vi "TagMetadataToImage.vi"(8 "error in (no error)":errorcluster, 10 "Image In":T1, 11 "LaserController in":refnum<class "LaserController.lvclass">) -> (0 "error out":errorcluster, 2 "Image Out":T1, 3 "LaserController out":refnum<class "LaserController.lvclass">)   [LabVIEW 2020, in "LaserController.lvlib" / "LaserController.lvclass"]
uses:
  LaserController.lvclass
  <vilib>/vision/Image Controls.llb/IMAQ Image.ctl
  LaserController.lvclass/LaserController.ctl
  Model/Hardware Abstraction Layer/Component/GenericActor/GenericActor/GenericController.lvclass
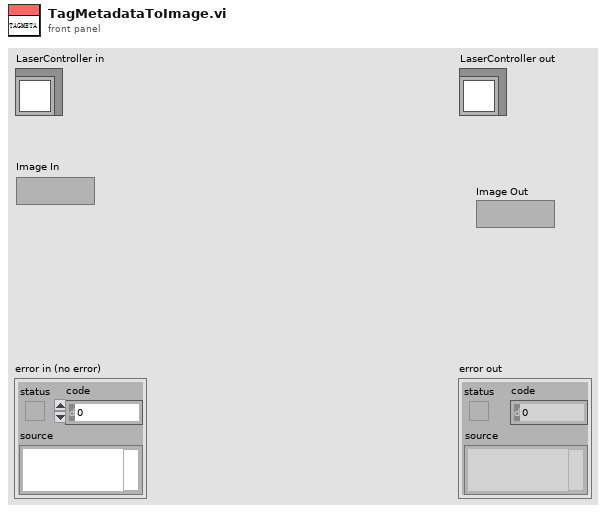
[diagram p1: front panel]
types:
  T1 = typedef "IMAQ Image.ctl" = refnum<image>
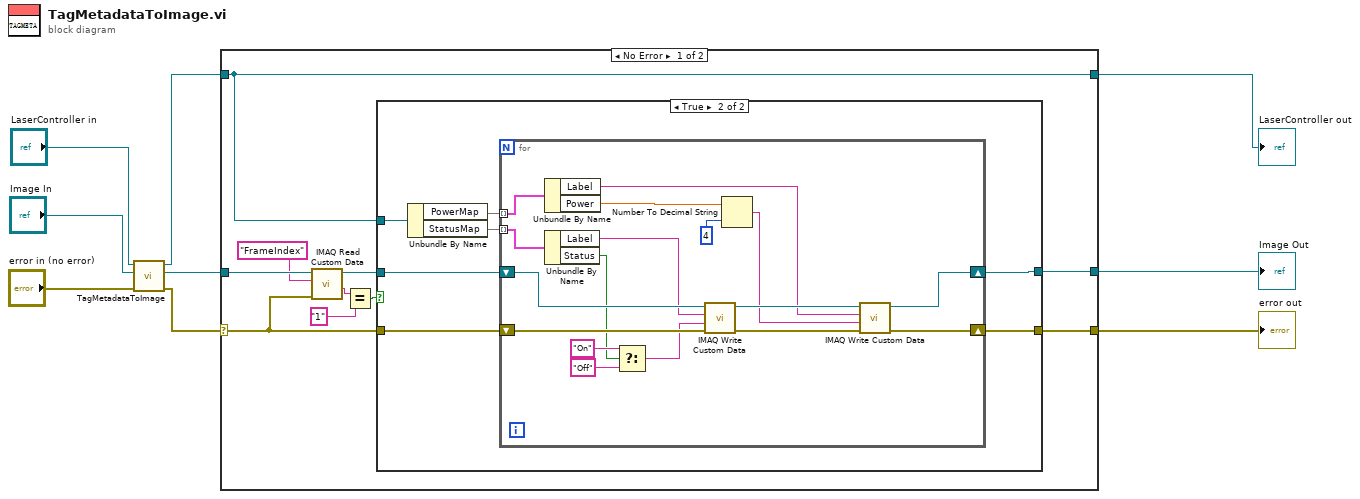
[diagram p0: block diagram]
diagram:
  n1 = call-parent "TagMetadataToImage.vi"("error in (no error)"="error in (no error)", "Image In"="Image In", "GenericController in"="LaserController in") -> ("error out"=w6:errorcluster, "Image Out"=w4:T1, "GenericController out"=w5:refnum<class "LaserController.lvclass">)  [unwired: 6 in]
  n2 = case shown="No Error" w6 {
    selector: w6 -> [w14 w48]
    tunnel: [w18 w48] -> w2
    tunnel: [w19 w47] -> w1
    tunnel: w5 -> [w19 w47]
    tunnel: w4 -> [w17 w46]
    tunnel: [w10 w46] -> w3
    frame No Error {
      n3 = call "IMAQ Read Custom Data"("error in (no error)"=w14, "Key"="FrameIndex", "Image"=w17) -> ("Custom Data Out"=w13:string, "Image (duplicate)"=w16:T1)  [unwired: 6 in, 1 out]
      n4 = Equal?(x=w13, y="1") -> (x = y?=w11:bool)
      n5 = case shown="True" w11 {
        tunnel: w19 -> [_ w28]
        tunnel: [w21 w27] -> w18
        tunnel: w16 -> [w20 w24]
        tunnel: w14 -> [w21 w23]
        tunnel: [w20 w22] -> w10
        frame False {
        }
        frame True {
          n6 = Unbundle By Name(w28) -> ("PowerMap"=w25:map{string, dbl}, "StatusMap"=w26:map{string, bool})
          n7 = for {
            shift-right: [w42] -> w27
            shift-left: w23 -> [w45]
            tunnel: w26 -> [w38] mode=indexing
            tunnel: w25 -> [w39] mode=indexing
            shift-right: [w40] -> w22
            shift-left: w24 -> [w43]
            n8 = Unbundle By Name(w39) -> ("Label"=w32:string, "Power"=w31:dbl)
            n9 = Unbundle By Name(w38) -> ("Label"=w37:string, "Status"=w34:bool)
            n10 = Select(t="On" ("y"), s=w34, f="Off" ("y")) -> (s? t:f=w33:string)
            n11 = call "IMAQ Write Custom Data"("error in (no error)"=w45, "Custom Data In"=w33, "Key"=w37, "Image"=w43) -> ("error out"=w44:errorcluster, "Image Out"=w41:T1)  [unwired: 6 in]
            n12 = Number To Decimal String(number=w31, width (-)=i16 4) -> (decimal integer string=w29:string)
            n13 = call "IMAQ Write Custom Data"("error in (no error)"=w44, "Custom Data In"=w29, "Key"=w32, "Image"=w41) -> ("error out"=w42:errorcluster, "Image Out"=w40:T1)  [unwired: 6 in]
          }
        }
      }
    }
    frame Error {
    }
  }
  "error out" <- w2
  "LaserController out" <- w1
  "Image Out" <- w3
